vi "NI-DAQmx.vi"() -> (0 "error out":errorcluster)   [LabVIEW 2022 SP3]
uses:
  Sub_vis/Upload Data.ctl
  5b8cb71c-e545-4ba2-a204-efceee465973.vi
  <vilib>/DAQmx/read.llb/DAQmx Read (Analog 2D DBL NChan NSamp).vi
  Globals/Meas_global.vi
  <vilib>/DAQmx/create/channels.llb/DAQmx Create Channel (AI-Voltage-Basic).vi
  <vilib>/DAQmx/configure/timing.llb/DAQmx Timing (Sample Clock).vi
  <vilib>/DAQmx/configure/trigger.llb/DAQmx Start Trigger (Digital Edge).vi
  <vilib>/DAQmx/miscellaneous.llb/DAQmx Fill In Error Info.vi
  <resource>/objmgr/daqmx.rc
  PWA/PWAtasksGLOBAL.vi
panel:
  out "errorLog":cluster{"error out":errorcluster, string}[](array[cluster])
  out "bufferSizeAssigned":u32
  out "totalPlannedSamples":i32
  out "Requested No of blocks":i32
  out "Current Block No":i32
  out "FsReq":dbl
  out "FsRead":dbl format="%#_11g"
  out "input terminal configuration":i32(ring)=10106 items=["default"=-1, "RSE"=10083, "NRSE"=10078, "Differential"=10106, "Pseudodifferential"=12529]
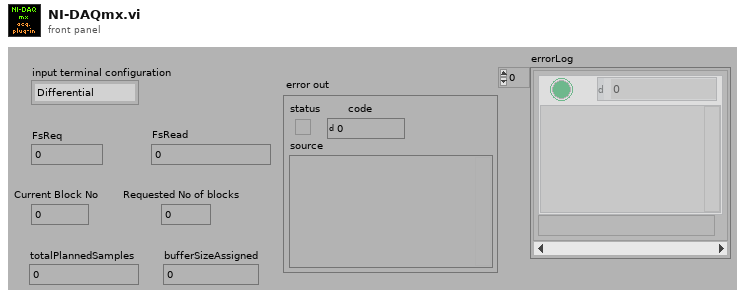
[diagram p1: front panel]
types:
  T1 = typedef "Analysis_info_cluster.ctl" = cluster{"Colour":u32, "Inst type":T2, "Inst name":string, "Symbol":string, "Code name":string, "Extra Info":string, "Inst Array":T3, "U":dbl, "u^2":dbl, "u^3":dbl, "u^4":dbl, "Skew_u":dbl, "Kurt_u":dbl, "Sd Error in Mean":dbl, "% u'/U":dbl, "X":dbl, "Y":dbl, "Z":dbl, "Timescale integral Estimate":dbl, "Sd Error in Variance":dbl, "Calib File":path, "Calib Constants":dbl[], "Output Position":bool, "Stats":enum16{"None", "Basic", "Full"}, "Av Sampling Rate":dbl, "Av No of Samples":dbl, "Total Meas Time (s)":dbl, "OrigChName":string, "Max value":dbl, "Min value":dbl, "Req Sample Rate Hz":dbl, "Sync Delay Time (s)":dbl, "Ch No":i16, "Device":string, "Use Latest Calib":bool, "Port":string, "Metadata Ch Names":string[], "Metadata Ch Values":string[], "Label":string, "chState":T4, "Point Drift":dbl, "inputConfig":string}
  T2 = typedef "Inst_type.ctl" = enum16{"Raw voltage", "Raw with zero offsetting", "Propeller anemometer", "Pressure Transducer", "Pitot-static tube", "Hot wire", "Cross wire 1", "Cross wire 2", "Generic Linear", "Generic Polynomial", "Generic BackPoly", "Fast FID", "Thermocouple", "Cold wire", "Pulsed Wire", "LDA Vel", "LDA Tran time", "LDA Arr time", "Microphone"}
  T3 = typedef "Instrument_Array.ctl" = enum16{"PWA", "LDA", "Analogue"}
  T4 = typedef "channelState.ctl" = enum32{"No Selection", "Solo", "Mute"}
  T5 = typedef "Device ID port info.ctl" = cluster{"Ch No":i16[], "Req Sampling Rate":dbl[], "Port":string, "Index":i32[]}
  T6 = typedef "Trigger_Mode.ctl" = enum16{"Free Running", "Start on Trigger", "Trigger Every Block", "Trigger Every Sample"}
  T7 = typedef "Upload Data.ctl" = enum16{"Voltage Array", "Time Trace Cluster"}
  T8 = typedef "Setup.ctl" = enum16{"Run Program", "Show Setup", "Save Current Setup", "Setup Front Panel"}
  T9 = typedef "Rendezvous RefNum" = refnum<k1>
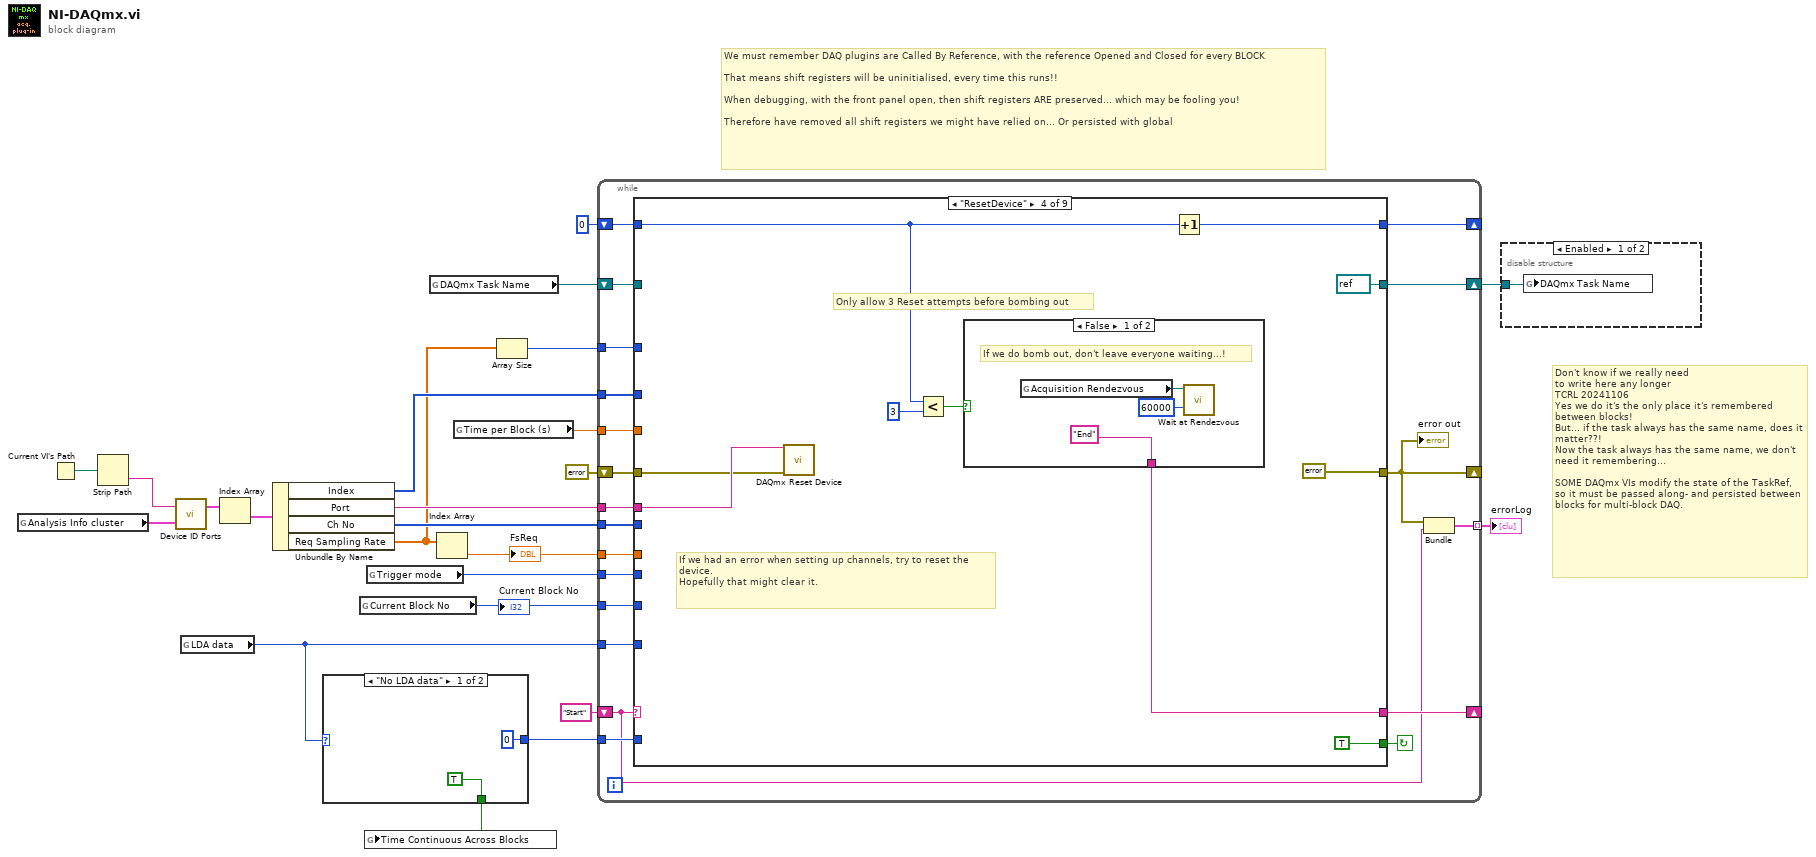
[diagram p0: block diagram]
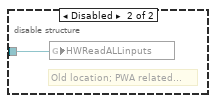
[diagram p2: hidden frame]
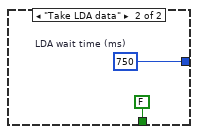
[diagram p3: hidden frame]
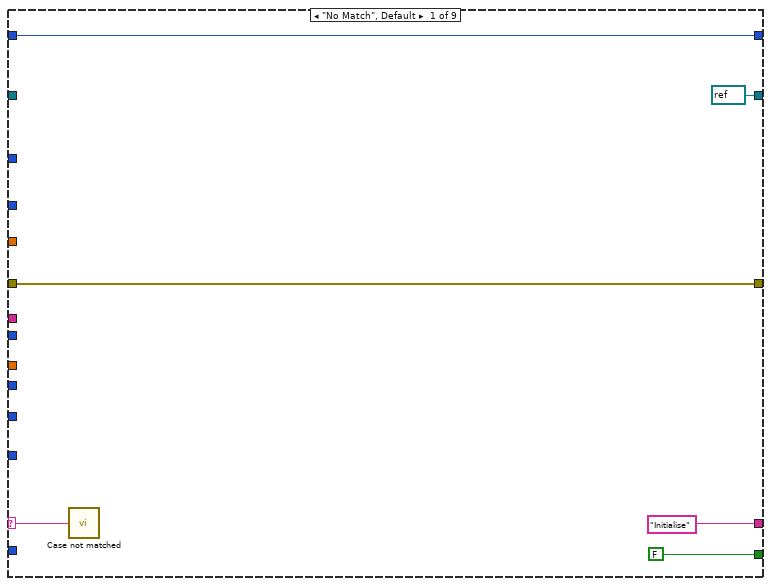
[diagram p4: hidden frame]
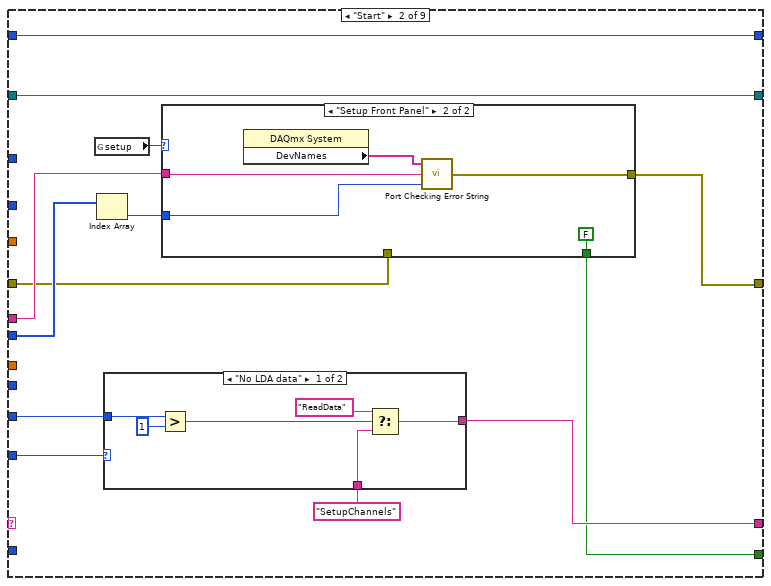
[diagram p5: hidden frame]
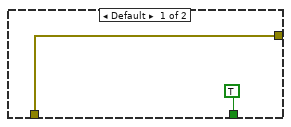
[diagram p6: hidden frame]
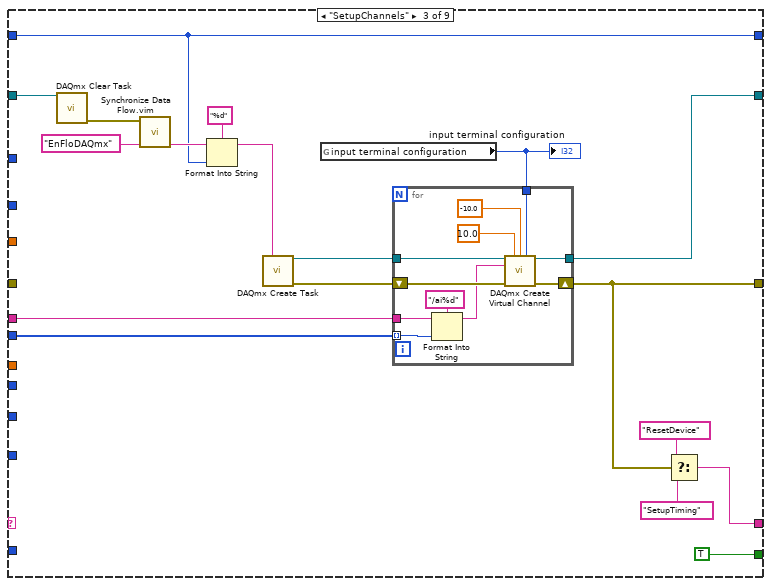
[diagram p8: hidden frame]
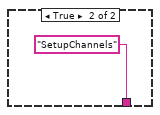
[diagram p9: hidden frame]
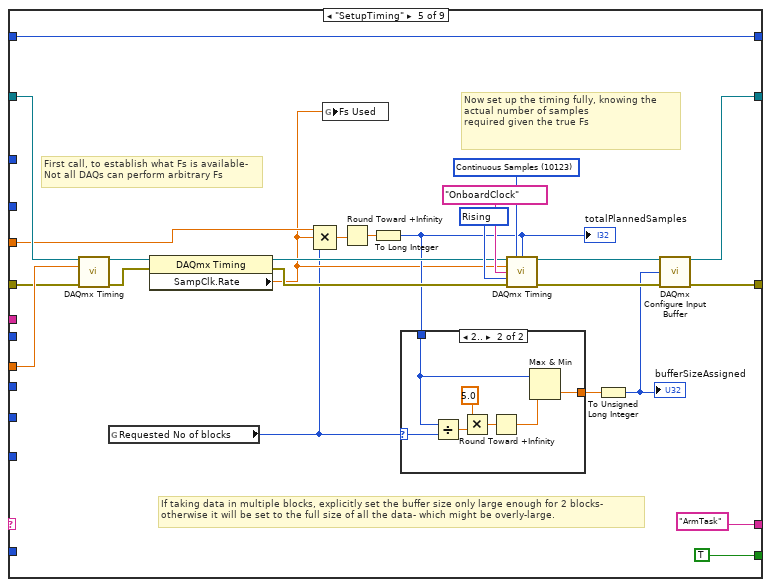
[diagram p10: hidden frame]
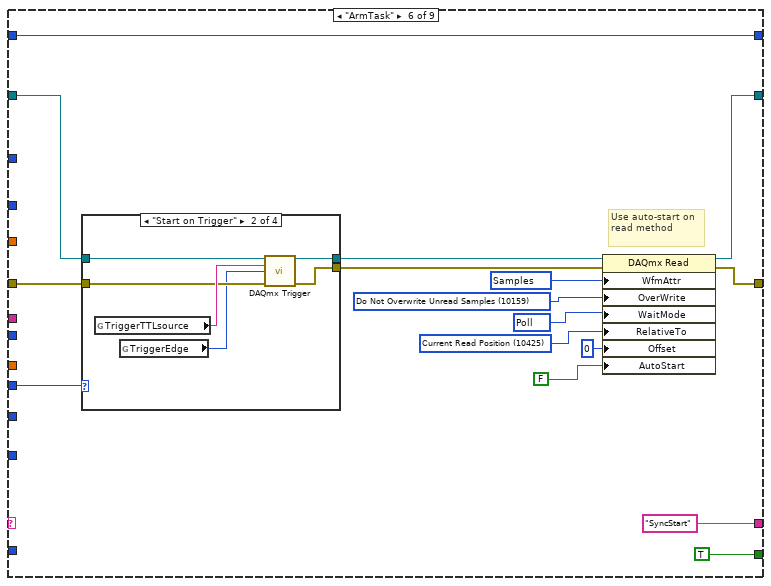
[diagram p12: hidden frame]
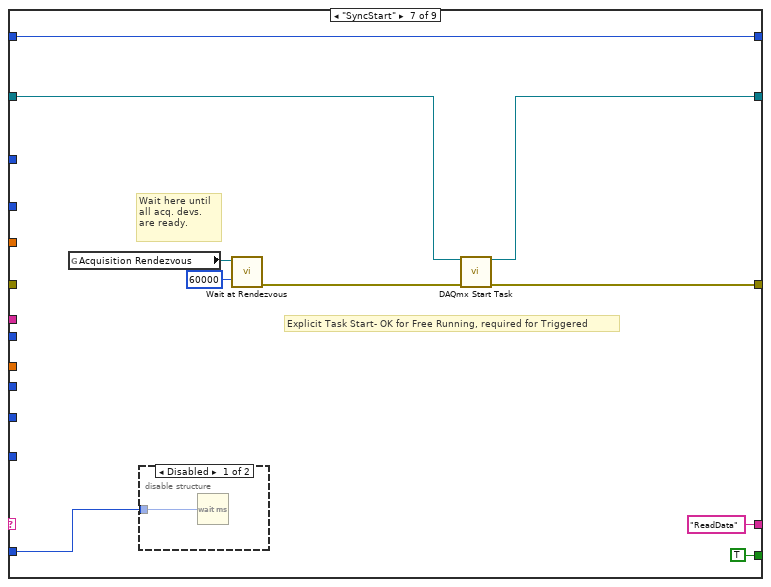
[diagram p16: hidden frame]
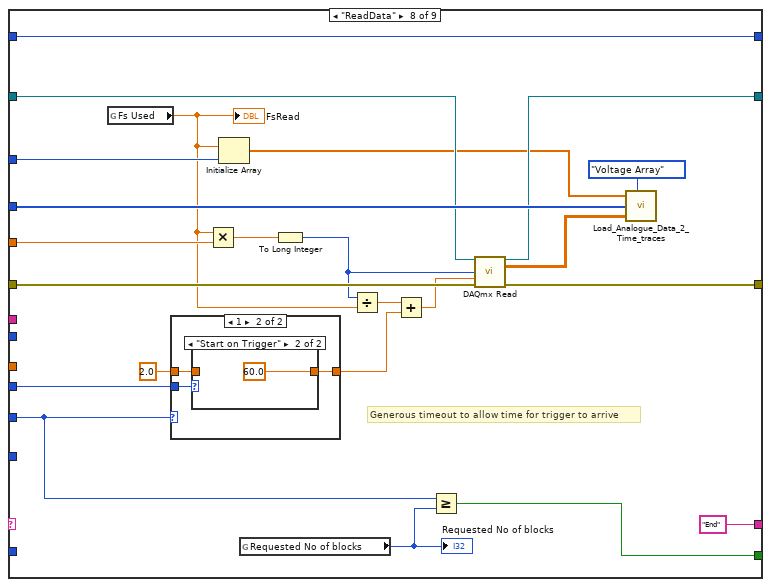
[diagram p18: hidden frame]
diagram:
  # "Don't know if we really need\nto write here any longer\nTCRL 20241106\nYes we do it's the only place it's remembered between blocks!\nBut... if the task always has the same name, does it matter??!\nNow the task always has the same name, we don't need it remembering...\n\nSOME DAQmx VIs modify the state of the TaskRef, so it must be passed along- and persisted between blocks for multi-block DAQ."
  # "We must remember DAQ plugins are Called By Reference, with the reference Opened and Closed for every BLOCK\n\nThat means shift registers will be uninitialised, every time this runs!!\n\nWhen debugging, with the front panel open, then shift registers ARE preserved... which may be fooling you!\n\nTherefore have removed all shift registers we might have relied on... Or persisted with global"
  n1 = global read "Meas_global.vi" "Analysis Info cluster"() -> (w12:T1[])
  n2 = Current VI's Path() -> (path=w19:path)
  n3 = Strip Path(path=w19) -> (name=w13:string)  [unwired: 1 out]
  n4 = call "Device ID Ports.vi"("Analysis Info cluster"=w12, "DAQdeviceType"=w13) -> ("Device port info"=w18:T5[])  [unwired: 1 out]
  n5 = global read "Meas_global.vi" "LDA data"() -> (w22:enum16{"No LDA data", "Take LDA data"})
  n6 = Index Array(array=w18) -> (element=w17:T5)  [unwired: 1 in]
  n7 = Unbundle By Name(w17) -> ("Index"=w15:i32[], "Port"=w16:string, "Ch No"=w14:i16[], "Req Sampling Rate"=w8:dbl[])
  n8 = case shown="\"No LDA data\"" w22 {
    tunnel: [TRUE ("Time Continuous across Blocks") FALSE ("Time Continuous across Blocks")] -> w21
    tunnel: [u32 0 ("LDA wait time (ms)") w26] -> w20
    frame "No LDA data" {
    }
    frame "Take LDA data" {
      w26 = u32 750  # LDA wait time (ms)
    }
  }
  n9 = global read "Meas_global.vi" "Current Block No"() -> (w10:i32)
  "Current Block No" <- w10
  n10 = global write "Meas_global.vi" "Time Continuous Across Blocks"(w21) -> ()
  n11 = global read "Meas_global.vi" "Trigger mode"() -> (w4:T6)
  n12 = global read "Meas_global.vi" "DAQmx Task Name"() -> (w3:refnum<k21>)
  n13 = Index Array(array=w8) -> (element=w7:dbl)  [unwired: 1 in]
  "FsReq" <- w7
  n14 = global read "Meas_global.vi" "Time per Block (s)"() -> (w11:dbl)
  n15 = Array Size(array=w8) -> (size(s)=w9:i32)
  n16 = while {
    shift-left: "Start" -> [w29]
    shift-right: [w33] -> _
    shift-right: [w30] -> _
    shift-left: errorcluster {"status"=FALSE, "code"=0, "source"=""} ("error out") -> [w34]
    tunnel: w7 -> [w47]
    tunnel: w10 -> [w46]
    shift-right: [w45] -> _
    shift-left: 0 -> [w44]
    tunnel: w22 -> [w43]
    tunnel: w20 -> [w42]
    tunnel: w14 -> [w41]
    tunnel: w16 -> [w40]
    tunnel: w15 -> [w39]
    tunnel: w11 -> [w37]
    tunnel: w9 -> [w35]
    tunnel: w4 -> [w32]
    shift-right: [w31] -> w2
    shift-left: w3 -> [w36]
    tunnel: [w28] -> w1 mode=indexing
    stop <- w38 continue-if-true
    n17 = case shown="\"ResetDevice\"" w29 {
      selector: w29 -> [w49 _ _ _ _ _ _ _ _]
      tunnel: [FALSE w57 TRUE TRUE TRUE TRUE TRUE w211 FALSE] -> w38
      tunnel: ["Initialise" w66 w90 w111 "ArmTask" "SyncStart" "ReadData" ("f") "End" "Start" ("f")] -> w33
      tunnel: [w51 w58 w92 errorcluster {"status"=FALSE, "code"=0, "source"=""} ("error out") w131 w169 w188 w214 w230] -> w30
      tunnel: w34 -> [w51 w56 _ w117 w143 w161 _ w218 w227]
      tunnel: w47 -> [_ _ _ _ w145 _ _ _ _]
      tunnel: w46 -> [_ w64 _ _ _ _ _ w207 _]
      tunnel: [w50 w65 w82 w114 w146 w170 w191 w216 w231] -> w45
      tunnel: w44 -> [w50 w65 w82 w118 w146 w170 w191 w216 w231]
      tunnel: w43 -> [_ w63 _ _ _ _ _ _ _]
      tunnel: w42 -> [_ _ _ _ _ _ w189 _ _]
      tunnel: w41 -> [_ w60 w95 _ _ _ _ _ _]
      tunnel: w40 -> [_ w61 w94 w119 _ _ _ _ _]
      tunnel: w39 -> [_ _ _ _ _ _ _ w215 _]
      tunnel: w37 -> [_ _ _ _ w128 _ _ w213 _]
      tunnel: w36 -> [_ w55 w87 _ w144 w162 w190 w209 w226]
      tunnel: w35 -> [_ _ _ _ _ _ _ w212 _]
      tunnel: w32 -> [_ _ _ _ _ w160 _ w208 _]
      tunnel: [refnum<k21> refnum ("task out") w55 w86 refnum<k21> refnum ("task out") w124 w158 w187 w206 refnum<k21> refnum ("task out")] -> w31
      frame "No Match", Default {
        n18 = call "Case not matched.vi"("Case Name not Matched"=w49) -> ()
      }
      frame "Start" {
        n19 = global read "Meas_global.vi" "setup"() -> (w62:T8)
        n20 = Index Array(array=w60) -> (element=w59:i16)  [unwired: 1 in]
        n21 = case shown="\"No LDA data\"" w63 {
          tunnel: [w79 w80] -> w66
          tunnel: w64 -> [w78 _]
          tunnel: "SetupChannels" -> [w74 w80]
          frame "No LDA data" {
            n22 = Greater?(x=w78, y=1) -> (0:w76:bool)
            n23 = Select(t="ReadData" ("f"), s=w76, f=w74) -> (s? t:f=w79:string)
          }
          frame "Take LDA data" {
          }
        }
        n24 = case shown="\"Setup Front Panel\"" w62 {
          tunnel: w61 -> [_ w72]
          tunnel: w59 -> [_ w73]
          tunnel: [w67 w71] -> w58
          tunnel: [TRUE FALSE] -> w57
          tunnel: w56 -> [w67 _]
          frame Default {
          }
          frame "Setup Front Panel" {
            n25 = property class="DAQmx System"() -> ("DevNames"=w69:tag[])  [unwired: 2 in, 2 out]
            n26 = call "Port Checking Error String.vi"("Ch Index"=w73, "Port"=w72, "Available Ports"=w69) -> ("error out"=w71:errorcluster)  [unwired: 1 in]
          }
        }
      }
      frame "SetupChannels" {
        n27 = call <vilib>:"DAQmx Clear Task.vi"("task in"=w87) -> ("error out"=w88:errorcluster)  [unwired: 14 in]
        n28 = call "Synchronize Data Flow.vim"("input 4"="EnFloDAQmx" ("new task name"), "input 1"=w88) -> ("output 4"=w84:string)  [unwired: 2 in, 3 out]
        n29 = Format Into String(format string="%d", initial string=w84, w82) -> (resulting string=w83:string)  [unwired: 1 in, 1 out]
        n30 = call <vilib>:"DAQmx Create Task.vi"("new task name"=w83) -> ("task out"=w97:refnum<k21>, "error out"=w98:errorcluster)  [unwired: 4 in, 9 out]
        n31 = global read "Meas_global.vi" "input terminal configuration"() -> (w93:i32)
        "input terminal configuration" <- w93
        n32 = for {
          shift-right: [w106] -> w92
          shift-left: w98 -> [w107]
          tunnel: w95 -> [w103] mode=indexing
          tunnel: w94 -> [w102]
          tunnel: w93 -> [w99]
          tunnel: w97 -> [w109]
          tunnel: [w108] -> w86
          n33 = Format Into String(format string="/ai%d", initial string=w102, w103) -> (resulting string=w104:string)  [unwired: 1 in, 1 out]
          n34 = call-poly <vilib>:"DAQmx Create Virtual Channel.vi"("task in"=w109, "maximum value"=10.0, "minimum value"=-10.0, "input terminal configuration"=w99, "physical channels"=w104, "error in"=w107) -> ("task out"=w108:refnum<k21>, "error out"=w106:errorcluster)  [unwired: 3 in, 5 out]
        }
        n35 = Select(t="ResetDevice", s=w92, f="SetupTiming") -> (s? t:f=w90:string)
      }
      frame "ResetDevice" {
        # "Only allow 3 Reset attempts before bombing out"
        # "If we had an error when setting up channels, try to reset the device.\nHopefully that might clear it."
        n36 = call <vilib>:"DAQmx Reset Device.vi"("device in"=w119, "error in"=w117) -> ()  [unwired: 13 in, 1 out]
        n37 = Less?(x=w118, y=3) -> (x < y?=w115:bool)
        n38 = case shown="False" w115 {
          tunnel: ["End" "SetupChannels"] -> w111
          frame False {
            # "If we do bomb out, don't leave everyone waiting...!"
            n39 = global read "Meas_global.vi" "Acquisition Rendezvous"() -> (w122:T9)
            n40 = call <vilib>:"Wait at Rendezvous.vi"("ms timeout (-1)"=60000, "rendezvous"=w122) -> ()  [unwired: 3 in, 3 out]
          }
          frame True {
          }
        }
        n41 = Increment(x=w118) -> (x+1=w114:i32)
      }
      frame "SetupTiming" {
        w139 = 10280 items=["Rising"=10280, "Falling"=10171] ("active edge")
        w141 = 10123 items=["Finite Samples"=10178, "Continuous Samples"=10123, "Hardware Timed Single Point"=12522] ("sample mode")
        # "If taking data in multiple blocks, explicitly set the buffer size only large enough for 2 blocks-\notherwise it will be set to the full size of all the data- which might be overly-large."
        # "Now set up the timing fully, knowing the actual number of samples\nrequired given the true Fs"
        # "First call, to establish what Fs is available-\nNot all DAQs can perform arbitrary Fs"
        n42 = call-poly <vilib>:"DAQmx Timing.vi"("task/channels in"=w144, "rate"=w145, "error in"=w143) -> ("task out"=w142:refnum<k21>, "error out"=w137:errorcluster)  [unwired: 4 in, 7 out]
        n43 = global read "Meas_global.vi" "Requested No of blocks"() -> (w125:i32)
        n44 = property class="DAQmx Timing"(reference=w142, error in=w137) -> (reference out=w138:refnum<k21>, error out=w136:errorcluster, "SampClk.Rate"=w127:dbl)
        n45 = Compound Arithmetic op=MULTIPLY(w128, w127, w125) -> (w126:dbl)
        n46 = global write "Meas_global.vi" "Fs Used"(w127) -> ()
        n47 = Round Toward +Infinity(x=w126) -> (ceil(x): smallest int >= x=w135:dbl)
        n48 = To Long Integer(number=w135) -> (32bit integer=w134:i32)
        "totalPlannedSamples" <- w134
        n49 = case shown="2.." w125 {
          selector: w125 -> [_ w154]
          tunnel: w134 -> [w149 w152]
          tunnel: [w149 w150] -> w130
          frame 1, Default {
          }
          frame 2.. {
            n50 = Divide(x=w152, y=w154) -> (x/y=w156:dbl)
            n51 = Multiply(x=5.0, y=w156) -> (x*y=w153:dbl)
            n52 = Round Toward +Infinity(x=w153) -> (ceil(x): smallest int >= x=w151:dbl)
            n53 = Max & Min(x=w152, y=w151) -> (min(x,y)=w150:dbl)  [unwired: 1 out]
          }
        }
        n54 = call-poly <vilib>:"DAQmx Timing.vi"("task/channels in"=w138, "sample mode"=w141, "samples per channel"=w134, "rate"=w127, "source"=tag "OnboardClock", "active edge"=w139, "error in"=w136) -> ("task out"=w132:refnum<k21>, "error out"=w133:errorcluster)  [unwired: 7 out]
        n55 = To Unsigned Long Integer(number=w130) -> (unsigned 32bit integer=w129:u32)
        "bufferSizeAssigned" <- w129
        n56 = call <vilib>:"DAQmx Configure Input Buffer.vi"("task/channels in"=w132, "buffer size (in samples per channel)"=w129, "error in"=w133) -> ("task out"=w124:refnum<k21>, "error out"=w131:errorcluster)  [unwired: 11 in]
      }
      frame "ArmTask" {
        w165 = 10425 items=["First Sample"=10424, "Current Read Position"=10425, "Reference Trigger"=10426, "First Pretrigger Sample"=10427, "Most Recent Sample"=10428] ("RelativeTo")
        w166 = 12524 items=["Wait For Interrupt"=12523, "Poll"=12524, "Yield"=12525, "Sleep"=12547] ("WaitMode")
        w167 = 10159 items=["Overwrite Unread Samples"=10252, "Do Not Overwrite Unread Samples"=10159] ("OverWrite")
        w168 = 10287 items=["Samples"=10287, "Samples and Timing"=10140, "Samples, Timing, and Attributes"=10141] ("WfmAttr")
        # "Use auto-start on read method"
        n57 = case shown="\"Start on Trigger\"" w160 {
          tunnel: [w173 w179 w181 w184] -> w163
          tunnel: w162 -> [w173 w178 w181 w184]
          tunnel: w161 -> [w174 w177 w182 w183]
          tunnel: [w174 w176 w182 w183] -> w159
          frame "Free Running", Default {
          }
          frame "Start on Trigger" {
            n58 = global read "Meas_global.vi" "TriggerTTLsource"() -> (w180:tag)
            n59 = global read "Meas_global.vi" "TriggerEdge"() -> (w175:i32)
            n60 = call-poly <vilib>:"DAQmx Trigger.vi"("task/channels in"=w178, "source"=w180, "edge"=w175, "error in"=w177) -> ("task out"=w179:refnum<k21>, "error out"=w176:errorcluster)  [unwired: 10 in]
          }
          frame "Trigger Every Block" {
          }
          frame "Trigger Every Sample" {
          }
        }
        n61 = property class="DAQmx Read"(reference=w163, error in=w159, "WfmAttr"=w168, "OverWrite"=w167, "WaitMode"=w166, "RelativeTo"=w165, "Offset"=0, "AutoStart"=FALSE) -> (reference out=w158:refnum<k21>, error out=w169:errorcluster)
      }
      frame "SyncStart" {
        # "Explicit Task Start- OK for Free Running, required for Triggered"
        # "Wait here until all acq. devs. are ready."
        n62 = global read "Meas_global.vi" "Acquisition Rendezvous"() -> (w193:T9)
        n63 = disable-structure shown="Disabled" {
          disable-tunnel: w189 -> [w195 _]
          frame Disabled {
            n64 = Wait (ms)(milliseconds to wait=w195) -> ()  [unwired: 1 out]
          }
          frame Enabled {
          }
        }
        n65 = call <vilib>:"Wait at Rendezvous.vi"("ms timeout (-1)"=60000, "rendezvous"=w193) -> ("error out"=w194:errorcluster)  [unwired: 3 in, 2 out]
        n66 = call <vilib>:"DAQmx Start Task.vi"("task/channels in"=w190, "error in"=w194) -> ("task out"=w187:refnum<k21>, "error out"=w188:errorcluster)  [unwired: 12 in]
      }
      frame "ReadData" {
        # "Generous timeout to allow time for trigger to arrive"
        n67 = global read "Meas_global.vi" "Fs Used"() -> (w198:dbl)
        "FsRead" <- w198
        n68 = case shown="1" w207 {
          tunnel: w208 -> [_ w222]
          tunnel: [w219 w221] -> w197
          tunnel: 2.0 ("y") -> [w219 w220]
          frame 2, Default {
          }
          frame 1 {
            n69 = case shown="\"Start on Trigger\"" w222 {
              tunnel: [w223 60.0 ("y")] -> w221
              tunnel: w220 -> [w223 _]
              frame "Free Running", Default {
              }
              frame "Start on Trigger" {
              }
            }
          }
        }
        n70 = Multiply(x=w198, y=w213) -> (x*y=w200:dbl)
        n71 = Initialize Array(w198, w212) -> (w202:dbl[])
        n72 = global read "Meas_global.vi" "Requested No of blocks"() -> (w210:i32)
        "Requested No of blocks" <- w210
        n73 = To Long Integer(number=w200) -> (32bit integer=w199:i32)
        n74 = Divide(x=w199, y=w198) -> (x/y=w205:dbl)
        n75 = Add(x=w205, y=w197) -> (x+y=w204:dbl)
        n76 = Greater Or Equal?(x=w207, y=w210) -> (x >= y?=w211:bool)
        n77 = call-poly <vilib>:"DAQmx Read.vi"("task/channels in"=w209, "number of samples per channel"=w199, "timeout"=w204, "error in"=w218) -> ("task out"=w206:refnum<k21>, "data"=w203:dbl[][], "error out"=w214:errorcluster)  [unwired: 9 out]
        n78 = call "Load_Analogue_Data_2_Time_traces.vi"("Sampling Rate (Hz)"=w202, "Mode"=Upload_Data."Voltage Array", "Index"=w215, "Voltage Array"=w203) -> ()  [unwired: 3 in]
      }
      frame "End" {
        n79 = call <vilib>:"DAQmx Stop Task.vi"("task/channels in"=w226, "error in"=w227) -> ("task out"=w229:refnum<k21>, "error out"=w228:errorcluster)  [unwired: 12 in]
        n80 = call <vilib>:"DAQmx Clear Task.vi"("task in"=w229, "error in"=w228) -> ("error out"=w230:errorcluster)  [unwired: 13 out]
      }
    }
    "error out" <- w30
    n81 = Bundle("error out"=w30, w29) -> (w28:cluster{"error out":errorcluster, string})  [unwired: 1 in]
  }
  "errorLog" <- w1
  n82 = disable-structure shown="Enabled" {
    disable-tunnel: w2 -> [w234 w235]
    frame Enabled {
      n83 = global write "Meas_global.vi" "DAQmx Task Name"(w234) -> ()
    }
    frame Disabled {
      # "Old location; PWA related..."
      n84 = global write "PWAtasksGLOBAL.vi" "HWReadALLinputs"(w235) -> ()
    }
  }
